vi "eventstruct.vi"() -> ()   [LabVIEW 2020]
panel:
  in  "String":string
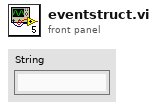
[diagram p1: front panel]
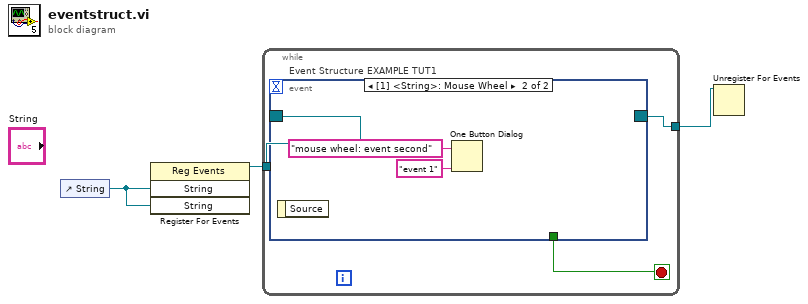
[diagram p0: block diagram]
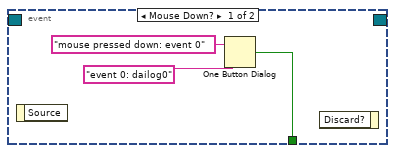
[diagram p2: hidden frame]
diagram:
  n1 = control-ref of="String"() -> (w1:refnum<vi>)
  n2 = register-events(w1, w1) -> (reference out=w3:refnum<event-registration>)  [unwired: 2 in, 1 out]
  n3 = while {
    tunnel: w3 -> [w6]
    tunnel: [w5] -> w2
    stop <- w4 stop-if-true
    n4 = event "Event Structure EXAMPLE TUT1" shown="[1] <String>: Mouse Wheel" {
      selector: w6 -> [_ _]
      dyn-events: [_ _] -> w5
      timeout: _ -> [_ _]
      tunnel: [w7 _] -> w4
      event Mouse Down? {
        n5 = event-data() -> ()  [unwired: 1 in, 1 out]
        n6 = One Button Dialog(message="mouse pressed down: event 0", button name ("OK")="event 0: dailog0") -> (true=w7:bool)
        n7 = event-data() -> ()  [unwired: 2 in, 1 out]
      }
      event Mouse Wheel {
        n8 = event-data() -> ()  [unwired: 1 in, 1 out]
        n9 = One Button Dialog(message="mouse wheel: event second", button name ("OK")="event 1") -> ()  [unwired: 1 out]
      }
    }
  }
  n10 = Unregister For Events(event registration refnum=w2) -> ()  [unwired: 1 in, 1 out]
